vi "RT Initialize Output Image (SubVI).vi"(8 "error in (no error)":errorcluster, 10 "Image Type":T1 items=["Grayscale (U8)", "Grayscale (I16)", "Grayscale (SGL)", "Complex (CSG)", "RGB (U32)", "HSL (U32)", "RGB (U64)", "Grayscale (U16)"], 11 "Image Size In":T3) -> (0 "error out":errorcluster, 3 "Output Image Out":T2)   [LabVIEW 2017, in "SoC IP Library.lvlib"]
uses:
  SoC IP Library.lvlib
  Controls/Image Size.ctl
  <vilib>/vision/Image Controls.llb/IMAQ Image.ctl
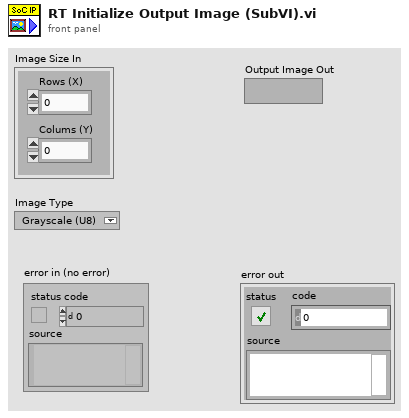
[diagram p1: front panel]
types:
  T1 = typedef "Image Type" = u32
  T2 = typedef "IMAQ Image.ctl" = refnum<image>
  T3 = typedef "SoC IP Library.lvlib/Image Size.ctl" = cluster{"Rows (X)":u16, "Colums (Y)":u16}
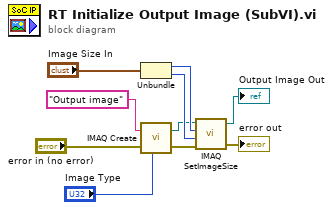
[diagram p0: block diagram]
diagram:
  n1 = Unbundle("Image Size In") -> ("Rows (X)"=w9:u16, "Colums (Y)"=w10:u16)
  n2 = call "IMAQ Create"("Image Name"="Output image", "Image Type"="Image Type", "error in (no error)"="error in (no error)") -> ("New Image"=w5:T2, "error out"=w4:errorcluster)  [unwired: 2 in]
  n3 = call "IMAQ SetImageSize"("error in (no error)"=w4, "Y Resolution"=w10, "X Resolution"=w9, "Image"=w5) -> ("error out"=→"error out":errorcluster, "Image Out"=→"Output Image Out":T2)  [unwired: 1 in]
